vi "Global 3.vi"() -> ()   [LabVIEW 2017]
panel:
  in  "Numeric":dbl
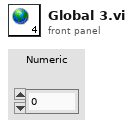
[diagram p1: front panel]
diagram:
